vi "GetFileVersionInfoSize.vi"(8 "error in (no error)":errorcluster, 11 "Path":path) -> (0 "error out":errorcluster, 2 "Size":i32, 3 "lptstrFilename":string)   [LabVIEW 2013, in "fileversion.lvlib"]
doc: "The GetFileVersionInfoSize function determines whether the operating system can retrieve version information for a specified file. If version information is available, GetFileVersionInfoSize returns the size, in bytes, of that information."
uses:
  fileversion.lvlib
  version.dll
panel:
  out "dummy lpdwHandle":i32
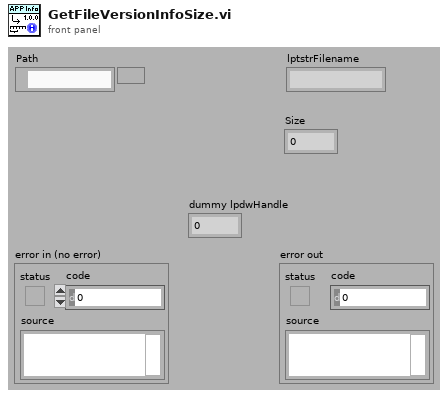
[diagram p1: front panel]
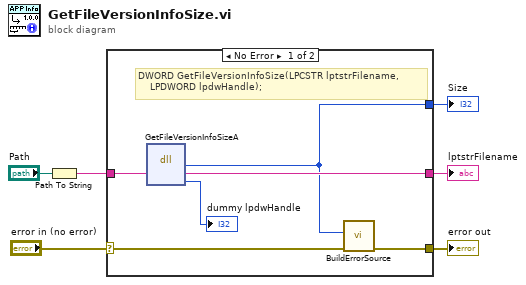
[diagram p0: block diagram]
diagram:
  n1 = Path To String(path="Path") -> (string=w1:string)
  n2 = case shown="No Error" "error in (no error)" {
    selector: "error in (no error)" -> [w9 w14]
    tunnel: [w8 w14] -> w6
    tunnel: [w12 w13] -> w5
    tunnel: [w7 _] -> w4
    tunnel: w1 -> [w10 w13]
    frame No Error {
      # "DWORD GetFileVersionInfoSize(LPCSTR lptstrFilename,\n    LPDWORD lpdwHandle);"
      n3 = dll-call lib="version.dll" fn="GetFileVersionInfoSizeA"("lptstrFilename"=w10) -> (w7:i32, "lptstrFilename"=w12:string, "lpdwHandle"=→"dummy lpdwHandle":i32)  [unwired: 4 in, 2 out]
      n4 = call "BuildErrorSource.vi"("error in"=w9, "status code"=w7) -> ("error out"=w8:errorcluster)  [unwired: 9 in]
    }
    frame Error {
    }
  }
  "error out" <- w6
  "lptstrFilename" <- w5
  "Size" <- w4
